vi "event.create_programmatic.vi"(4 "type":enum16{"INFO", "FLAG", "ERROR", "SUCCESS"}(ring), 5 "Duration (s)":dbl, 6 "Properties and Labels":T1, 7 "Time Stamp (now: system time)":timestamp format="%<%x %.3X>T", 8 "error in":errorcluster, 9 "Name":string, 10 "Asset RIDs":string[](array[string]), 11 "Nominal Client in":refnum<class "Nominal Client.lvclass">) -> (0 "error out":errorcluster, 3 "Nominal Client out":refnum<class "Nominal Client.lvclass">)   [LabVIEW 2020, in "Nominal Client.lvclass"]
doc: "Creates a timestamped event in Nominal associated with one or more assets, marking significant occurrences during test execution such as hardware state changes or sequence transitions. Events appear alongside telemetry data to enable correlation between test activities and system behavior during analysis."
uses:
  Nominal Client.lvclass
  Nominal Client.lvclass/Nominal Client.ctl
  00420838-c675-47b9-9aa3-23bdaed8b651.vi
  461845d9-5b01-42d7-9db3-adb116d554ee.vi
  bf5e2bc1-b739-4656-bb34-8a0d936475ea.vi
  10b04410-bb00-4972-b447-bcffff0721b9.vi
  d05a9046-6d13-4bf3-8ca7-a2c5711d0a3f.vi
  trace.payload_received.vi
  error.vi
  trace.payload_sent.vi
  create.authorization_header.vi
  trace.calling_method.vi
  error.vi/859f8e04-e495-489b-b5b4-7ac163f56130.vi
  <vilib>/JDP Science/JDP Science Common Utilities/Trim Whitespace__JDP.vi
  <vilib>/AdvancedString/1D String Array to Delimited String.vi
  api_token.get.vi
  <vilib>/LabVIEW Open Source Project/Epoch Date & Time/epoch.UNIX/Epoch.UNIX.lvclass
  C:/Program Files/National Instruments/LabVIEW 2020/vi.lib/LabVIEW Open Source Project/Epoch Date & Time/epoch/Epoch.lvclass
  <vilib>/LabVIEW Open Source Project/Epoch Date & Time/Get Epoch Time.vi
  <vilib>/JDP Science/JSONtext/Variant to JSON Text.vi
  <vilib>/JDP Science/JSONtext/support/Format JSON Object.vi
  <vilib>/Utility/libraryn.llb/Get File Extension.vi
  log_file.write.vi
  <vilib>/JDP Science/JSONtext/Get all Object Items.vi
  <vilib>/Utility/error.llb/Error Cluster From Error Code.vi
  <vilib>/JDP Science/JSONtext/JSON text to Variant.vi
  <vilib>/JDP Science/JSONtext/LVClass Serializer/JSONtext LVClass Serializer.lvclass
  <vilib>/addons/_JKI.lib/REST Client/classes/Response Headers/Response Headers.lvclass
  nominal types/properties/properties.lvclass
  nominal types/labels/labels.lvclass
  <vilib>/addons/_JKI.lib/REST Client/classes/REST Client/REST Client.lvclass
  <vilib>/JDP Science/JSONtext/JSONtext.lvlib
  29b9c2c3-1894-4cda-8e40-3f5b7728bbf5.vi
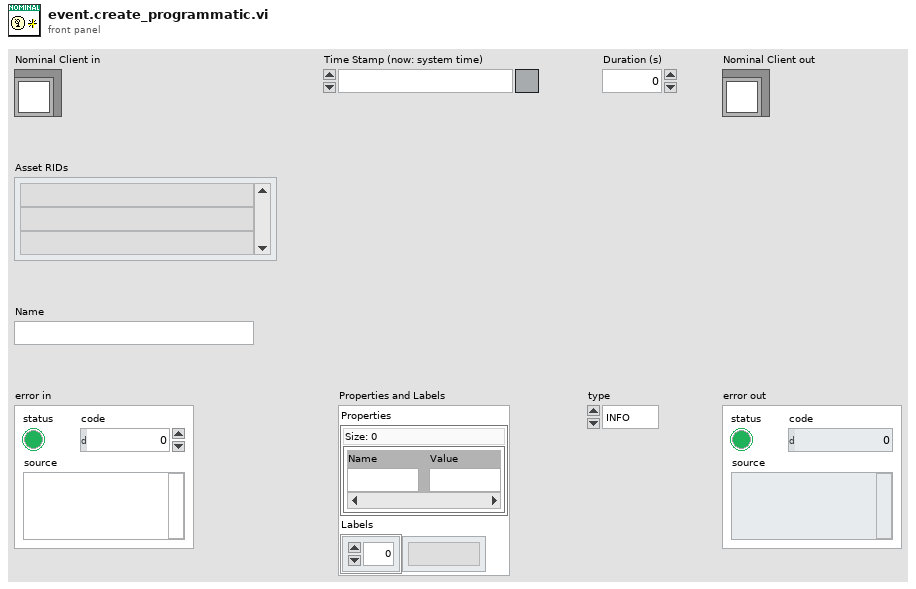
[diagram p1: front panel]
types:
  T1 = cluster{"Properties":map{string, string}, "Labels":string[]}
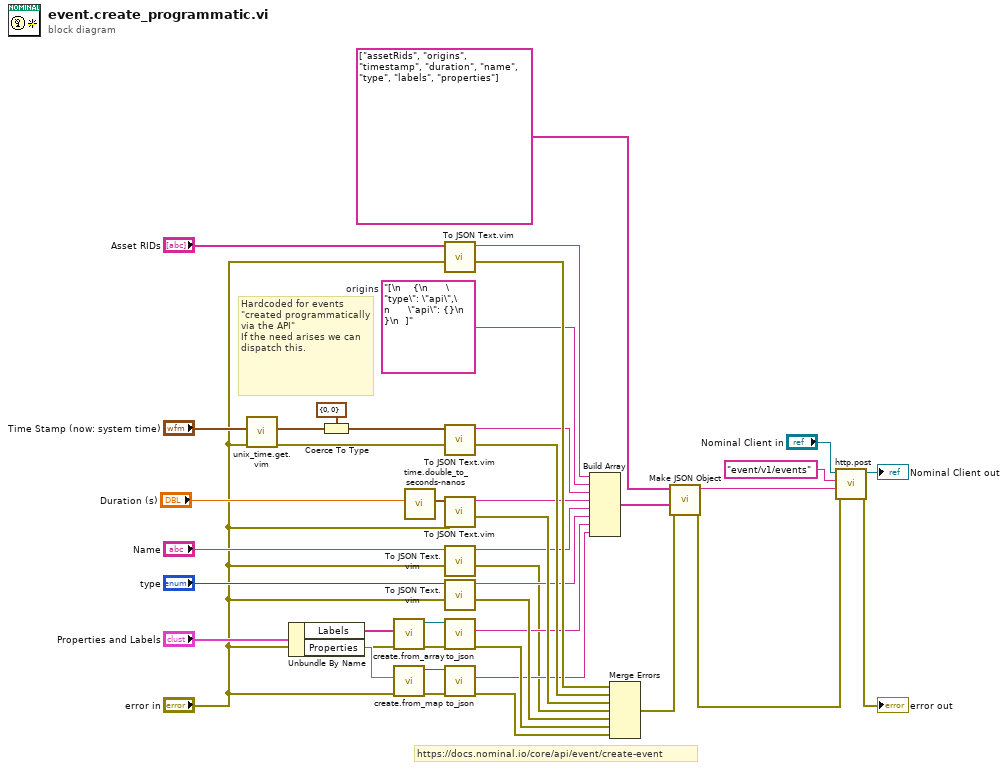
[diagram p0: block diagram]
diagram:
  w18 = "[\n    {\n      \"type\": \"api\",\n      \"api\": {}\n    }\n  ]"  # origins
  # "Hardcoded for events \"created programmatically via the API\"\nIf the need arises we can dispatch this."
  # "https://docs.nominal.io/core/api/event/create-event"
  n1 = call "unix_time.get.vim"("Time Stamp (empty: now) [single or array]"="Time Stamp (now: system time)") -> ("UNIX Timestamp"=w40:cluster{"Seconds":i64, "Nanoseconds":i64})  [unwired: 10 in]
  n2 = Unbundle By Name("Properties and Labels") -> ("Labels"=w32:string[], "Properties"=w34:map{string, string})
  n3 = Coerce To Type(0:w40, 1:cluster{"seconds":i32, "nanos":i32} {"seconds"=0, "nanos"=0} ("UNIX Timestamp")) -> (2:w26:cluster{"seconds":i32, "nanos":i32})
  n4 = call "create.from_array.vi"("error in"="error in", "labels"=w32) -> ("error out"=w30:errorcluster, "labels out"=w31:refnum<class "labels.lvclass">)  [unwired: 8 in]
  n5 = call "create.from_map.vi"("error in"="error in", "properties"=w34) -> ("error out"=w29:errorcluster, "properties out"=w33:refnum<class "properties.lvclass">)  [unwired: 8 in]
  n6 = call "time.double_to_seconds-nanos.vi"("Time (s)"="Duration (s)") -> ("Seconds Nanos"=w4:cluster{"seconds":i32, "nanos":i32})  [unwired: 10 in]
  n7 = call "To JSON Text.vim"("error in (no error)"="error in", "Anything"="Asset RIDs") -> ("error out"=w23:errorcluster, "<JSON>"=w27:string)  [unwired: 8 in]
  n8 = call "To JSON Text.vim"("error in (no error)"="error in", "Anything"=w26) -> ("error out"=w22:errorcluster, "<JSON>"=w17:string)  [unwired: 8 in]
  n9 = call "To JSON Text.vim"("error in (no error)"="error in", "Anything"=w4) -> ("error out"=w41:errorcluster, "<JSON>"=w3:string)  [unwired: 8 in]
  n10 = call "To JSON Text.vim"("error in (no error)"="error in", "Anything"="Name") -> ("error out"=w1:errorcluster, "<JSON>"=w13:string)  [unwired: 8 in]
  n11 = call "To JSON Text.vim"("error in (no error)"="error in", "Anything"="type") -> ("error out"=w21:errorcluster, "<JSON>"=w16:string)  [unwired: 8 in]
  n12 = call-dynamic "to_json.vi"("error in"=w30, "labels in"=w31) -> ("error out"=w20:errorcluster, "json"=w15:string)  [unwired: 6 in, 2 out]
  n13 = call-dynamic "to_json.vi"("error in"=w29, "properties in"=w33) -> ("error out"=w19:errorcluster, "json"=w14:string)  [unwired: 6 in, 2 out]
  n14 = Build Array(w27, w18, w17, w3, w13, w16, w15, w14) -> (w25:string[])
  n15 = Merge Errors(w23, w22, w41, w1, w21, w20, w19) -> (w12:errorcluster)
  n16 = call <vilib>:"Make JSON Object.vi"("error in (no error)"=w12, "JSON Items"=w25, "Item Names"=string[] ["assetRids", "origins", "timestamp", "duration", "name", "type", "labels", "properties"]) -> ("error out"=w7:errorcluster, "<JSON>"=w6:string)  [unwired: 7 in]
  n17 = call "http.post.vi"("error in"=w7, "Request body"=w6, "Path"="event/v1/events", "Nominal Client in"="Nominal Client in") -> ("error out"=→"error out":errorcluster, "Nominal Client out"=→"Nominal Client out":refnum<class "Nominal Client.lvclass">)  [unwired: 4 in, 2 out]
